vi "Get Events.vi"(11 "Main View in":refnum<class "Main View.lvclass">) -> (2 "Events":T1, 3 "Main View out":refnum<class "Main View.lvclass">)   [LabVIEW 2013, in "Main View.lvlib" / "Main View.lvclass"]
uses:
  Main View.lvclass
  Typedef/Events.ctl
  Main View.lvclass/Main View.ctl
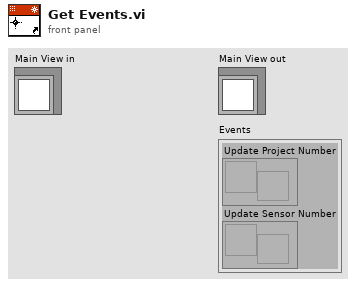
[diagram p1: front panel]
types:
  T1 = typedef "Main View.lvlib/Main View.lvclass/Events.ctl" = cluster{"Update Project Number":refnum<user-event>, "Update Sensor Number":refnum<user-event>}
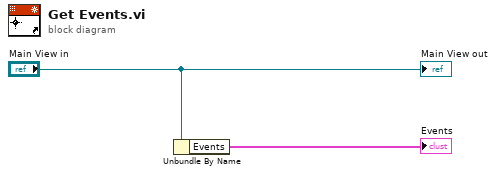
[diagram p0: block diagram]
diagram:
  n1 = Unbundle By Name("Main View in") -> ("Events"=→"Events":T1)
  "Main View out" <- "Main View in"
